vi "Check-displacement.vi"(8 "error in (no error)":errorcluster, 10 "Displacement in":dbl caption="Displacement [unit]", 11 "Motor-Serial in":refnum<class "Motor-Serial.lvclass">) -> (0 "error out":errorcluster, 1 "In range?":bool, 2 "Displacement out":dbl caption="Displacement out [unit]", 3 "Motor-Serial out":refnum<class "Motor-Serial.lvclass">)   [LabVIEW 2013, in "PowderDeposition.lvlib" / "Motor-Serial.lvclass"]
uses:
  Motor-Serial.lvclass
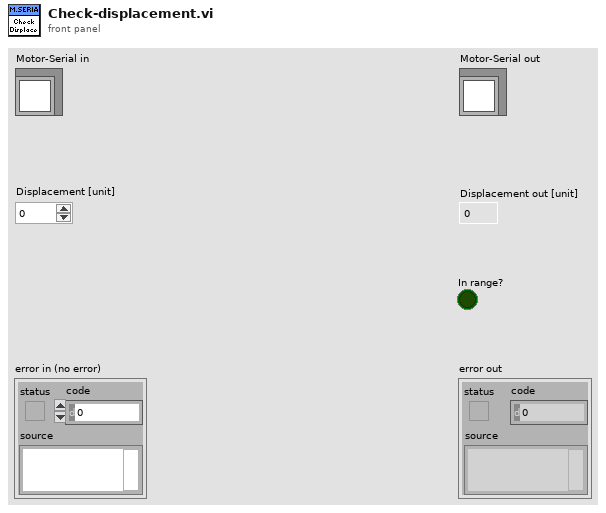
[diagram p1: front panel]
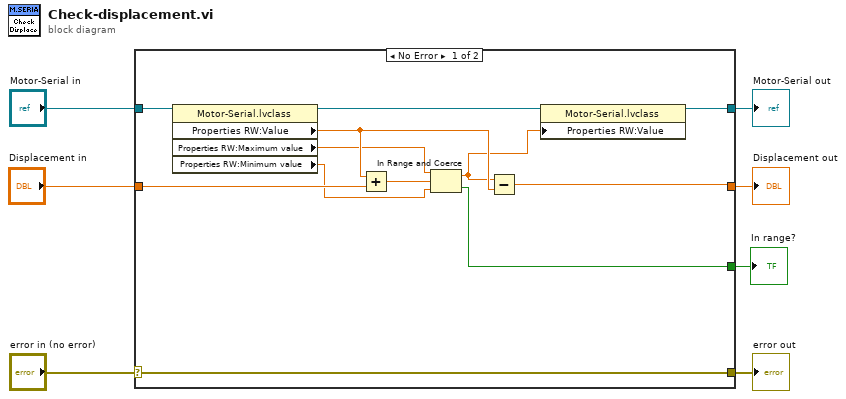
[diagram p0: block diagram]
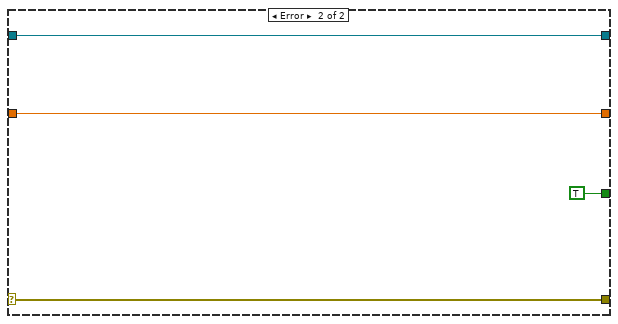
[diagram p2: hidden frame]
diagram:
  n1 = case shown="No Error" "error in (no error)" {
    selector: "error in (no error)" -> [w18 w23]
    tunnel: [w18 w23] -> w6
    tunnel: [w9 w22] -> w4
    tunnel: "Motor-Serial in" -> [w19 w22]
    tunnel: "Displacement in" -> [w16 w21]
    tunnel: [w14 w21] -> w2
    tunnel: [w10 TRUE] -> w1
    frame No Error {
      n2 = property class="Motor-Serial.lvclass"(reference=w19) -> (reference out=w17:refnum<class "Motor-Serial.lvclass">, "Properties RW:Value"=w15:dbl, "Properties RW:Maximum value"=w11:dbl, "Properties RW:Minimum value"=w12:dbl)  [unwired: 1 in, 1 out]
      n3 = Add(x=w15, y=w16) -> (x+y=w13:dbl)
      n4 = In Range and Coerce(upper limit=w11, x=w13, lower limit=w12) -> (coerced(x)=w8:dbl, In Range?=w10:bool)
      n5 = Subtract(x=w8, y=w15) -> (x-y=w14:dbl)
      n6 = property class="Motor-Serial.lvclass"(reference=w17, "Properties RW:Value"=w8) -> (reference out=w9:refnum<class "Motor-Serial.lvclass">)  [unwired: 1 in, 1 out]
    }
    frame Error {
    }
  }
  "error out" <- w6
  "Motor-Serial out" <- w4
  "Displacement out" <- w2
  "In range?" <- w1
